vi "clearpath_crio.vi"() -> ()   [LabVIEW 2010]
doc: "Overall demo interface for the cRIO implementation of the Clearpath Control Panel. Allows users to manually issue commands and request subscriptions to a variety of data messages."
uses:
  clearpath_interface.lvlib
panel:
  in  "Int Lim":dbl
  in  "Stic":dbl
  in  "FF":dbl
  in  "D":dbl
  in  "I":dbl
  in  "P":dbl
  in  "Set Controls":bool
  in  "Reset":bool
  in  "Remote E-Stop":bool
  in  "Set Safety":bool
  in  "New Chassis Time (ms)":u32
  in  "Set Time":bool
  in  "New Chassis Name":string
  in  "Set Name":bool
  in  "Max Accel":dbl
  in  "Set Max Accel":bool
  in  "Max Speed":dbl
  in  "Set Max Speed":bool
  in  "Right Accel":dbl
  in  "Left Accel":dbl
  in  "Command Repeat Period (ms)":i32=100
  in  "Continuous Speeds":bool
  in  "Left Speed":dbl
  in  "Right Speed":dbl
  in  "Set Speeds":bool
  in  "Continuous Output":bool
  in  "Left Output":dbl
  in  "Right Output":dbl
  in  "Set Output":bool
  in  "Update Safety Status":bool
  in  "FreqSafetyStatus":u8
  in  "Update Power System":bool
  in  "FreqPowerSystem":u8
  in  "Update Platform Rotation":bool
  in  "FreqPlatformRot":u8
  in  "Update System Status":bool
  in  "FreqSystemStatus":u8
  in  "Update Differential Speed":bool
  in  "FreqDifferentialSpeed":u8
  in  "Update Differential Output":bool
  in  "FreqDifferentialOutput":u8
  in  "Update Differential Control":bool
  in  "FreqDifferentialControl":u8
  in  "Update Platform Name":bool
  in  "FreqPlatformName":u8
  in  "Update Platform Info":bool
  in  "FreqPlatformInfo":u8
  in  "Update Max Accel":bool
  in  "FreqMaxAccel":u8
  in  "Update Max Speed":bool
  in  "FreqMaxSpeed":u8
  in  "Update Firmware Info":bool
  in  "FreqFirmwareInfo":u8
  in  "Update Raw Encoders":bool
  in  "FreqRawEncoder":u8
  in  "Set Brake":bool
  in  "Continuous Vel":bool
  in  "Translational Speed":dbl
  in  "Rotational Speed":dbl
  in  "Set Velocity":bool
  in  "Update Encoder":bool
  in  "FreqEncoder":u8
  in  "VISA resource name":refnum<visa-resource-name>="ASRL1::INSTR"
  in  "Baud rate":dbl=115200.0
  in  "stop":bool
  # "Communication Status"
  # "Subscriptions"
  # "Platform Info (0x8001)"
  # "Differential Control (0x8201)"
  # "Platform Name (0x8002)"
  # "Differential Output (0x8202)"
  # "Firmware Info (0x8003)"
  # "Max Speed (0x8210)"
  # "System Status (0x8004)"
  # "Max Accel (0x8211)"
  # "Power System (0x8005)"
  # "Platform Rotation (0x8601)"
  # "Safety System Status (0x8010)"
  # "Encoders (0x8800)"
  # "Differential Speed (0x8200)"
  # "Raw Encoders (0x8801)"
  # "Set Velocity"
  # "Set Differential Speeds"
  # "Set Chassis Name/Time"
  # "Set Differential Controls"
  # "Set Safety System"
  # "Set Differential Output"
  # "Set Max Speed/Accel"
  # "Reset Processor"
  # "Control Test Panel\nClearpath Control Protocol cRIO Test Interface v1.0\nClearpath Robotics Inc., (c) 2010"
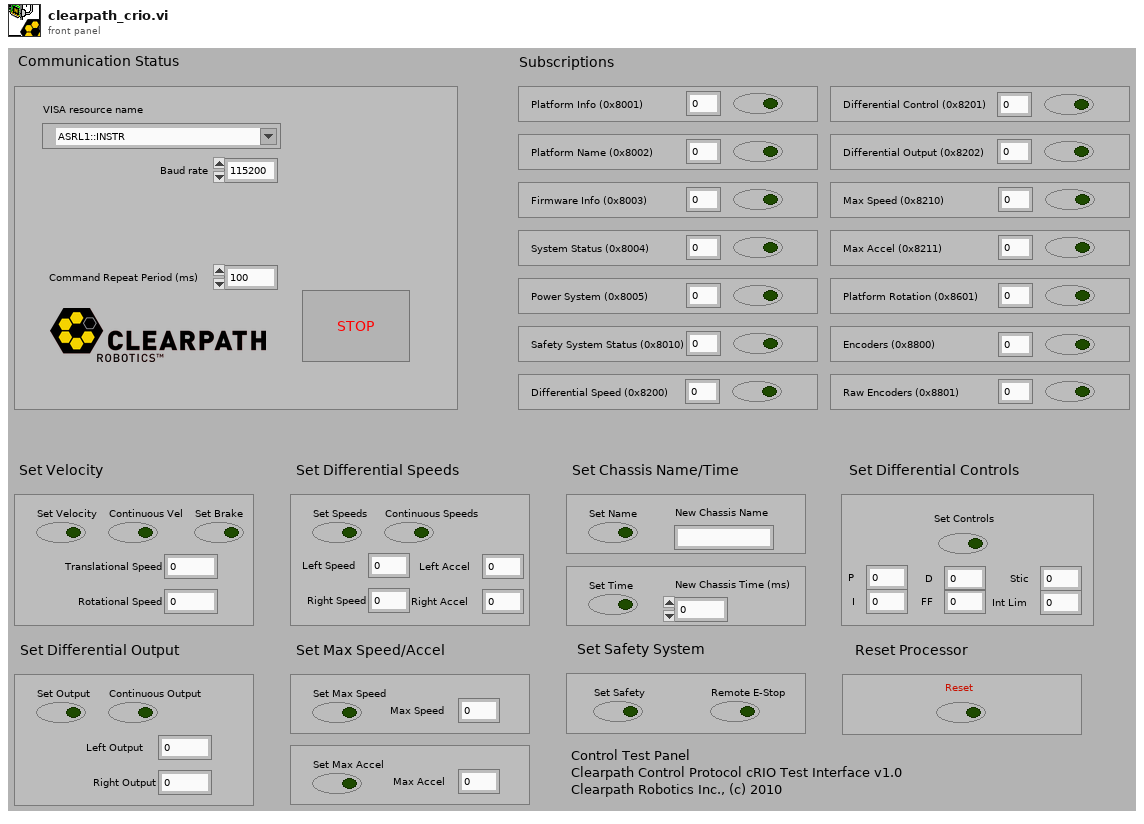
[diagram p1: front panel]
types:
  T1 = cluster{"Xmit Queue":refnum<queue>, "Data Queue":refnum<queue>, "VISA resource name out":refnum<visa-resource-name>, "error out":errorcluster, "Message Data Cluster":cluster{"\nChar Idx":u8, "Num. Char Rem":u8, "Write Index":u8, "Read Index":u8, "Message Data Buffer":u8[][]}}
  T2 = cluster{"P":dbl, "I":dbl, "D":dbl, "FF":dbl, "Stic":dbl, "Int Lim":dbl}
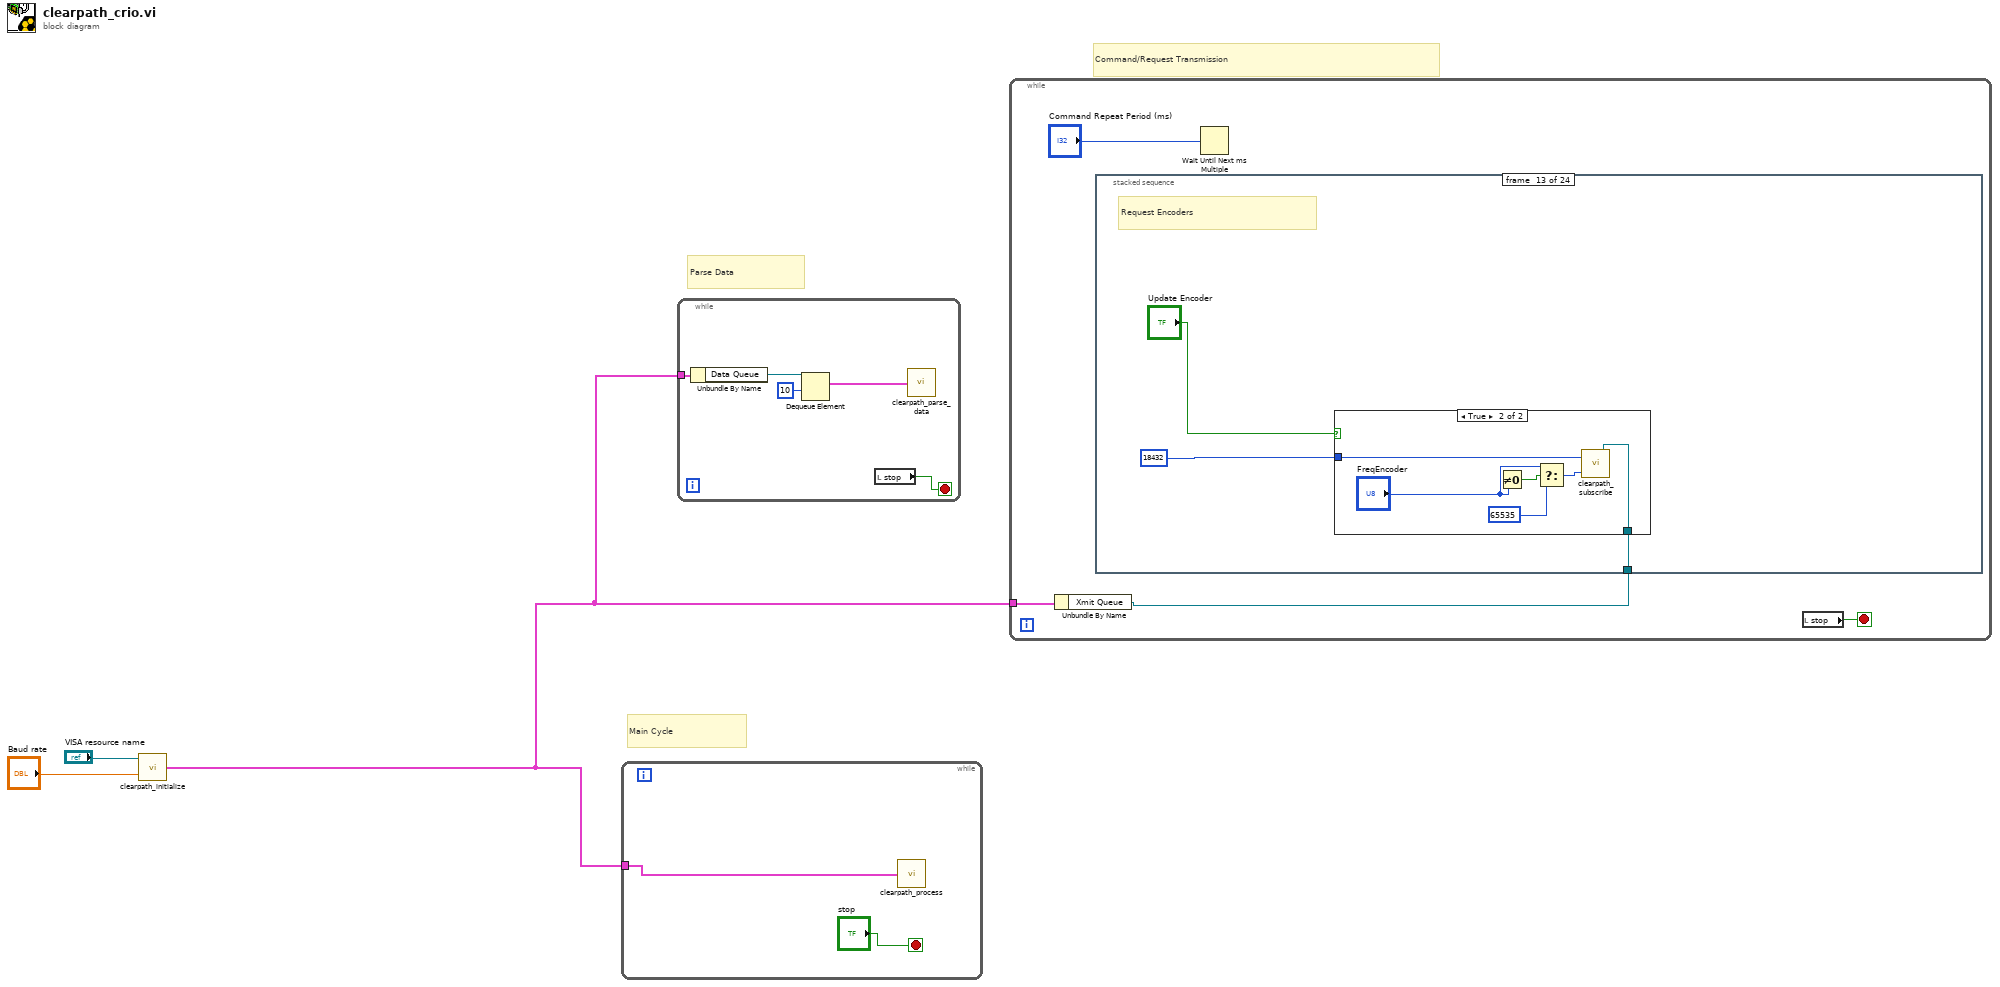
[diagram p0: block diagram]
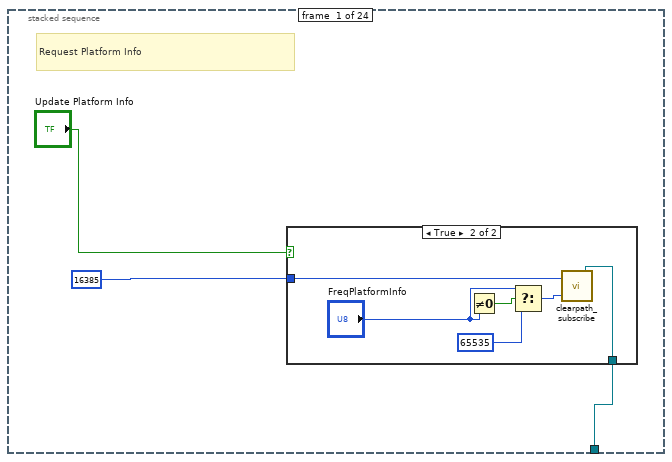
[diagram p2: hidden frame]
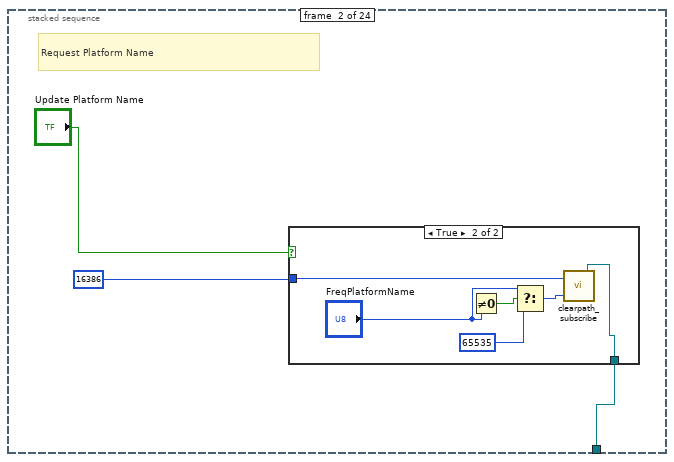
[diagram p4: hidden frame]
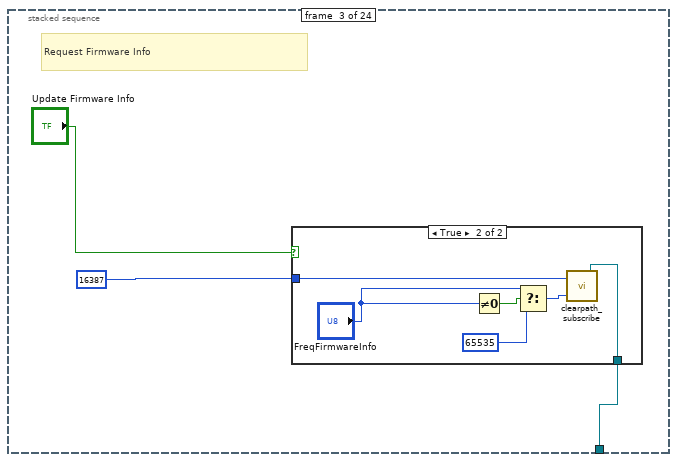
[diagram p6: hidden frame]
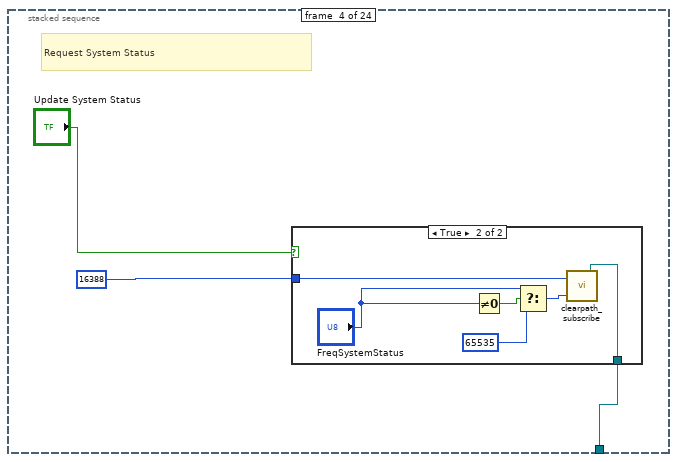
[diagram p8: hidden frame]
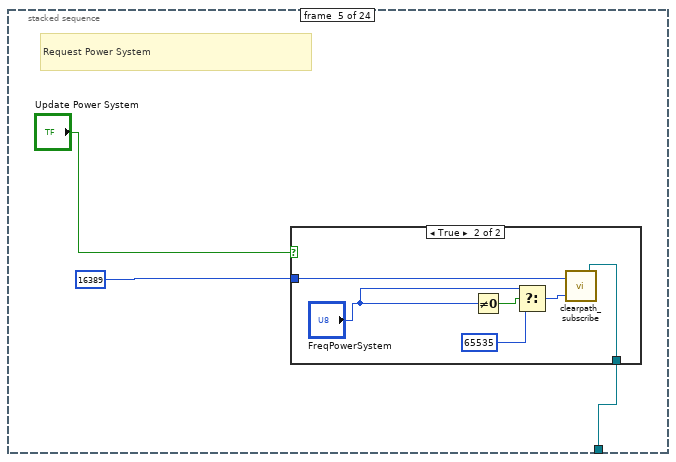
[diagram p10: hidden frame]
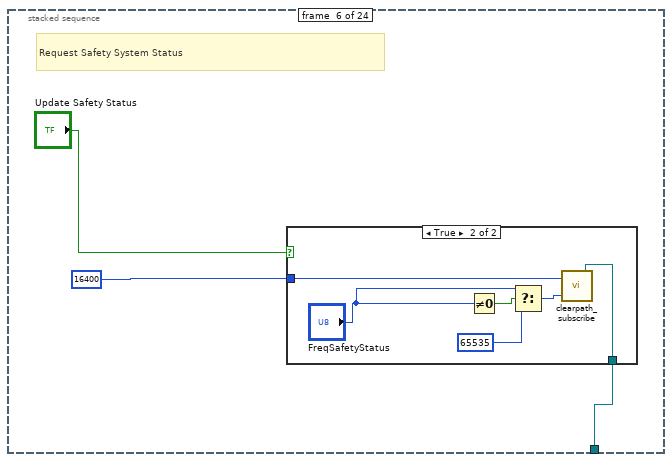
[diagram p12: hidden frame]
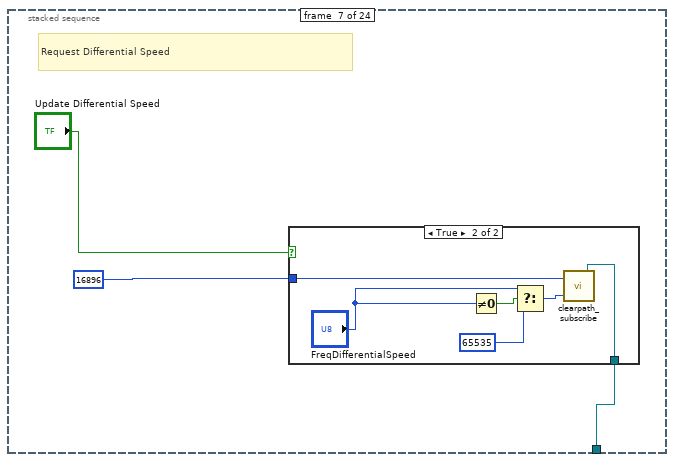
[diagram p14: hidden frame]
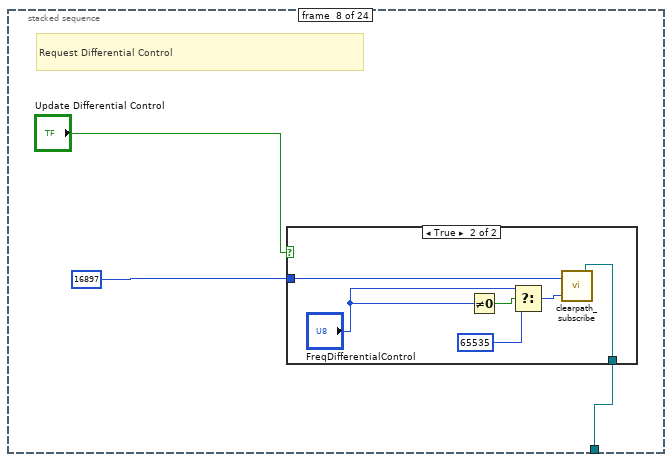
[diagram p16: hidden frame]
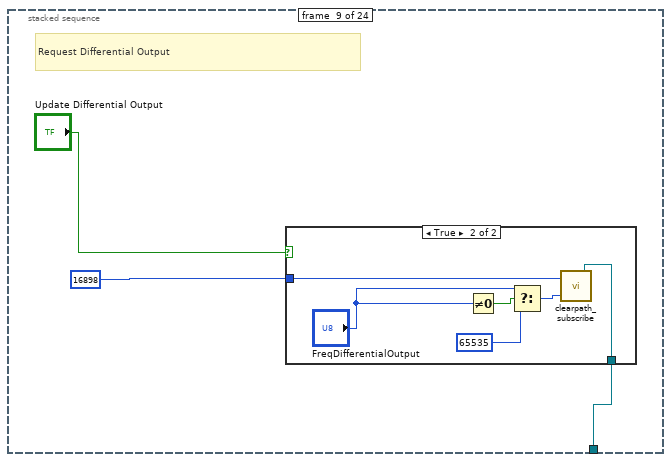
[diagram p18: hidden frame]
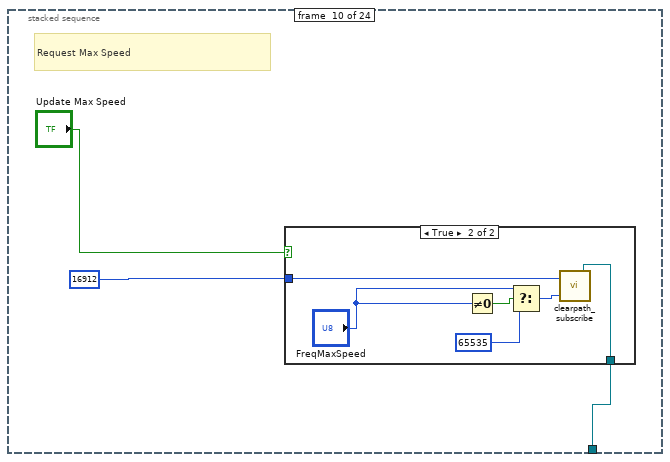
[diagram p20: hidden frame]
diagram:
  # "Main Cycle"
  # "Parse Data"
  # "Command/Request Transmission"
  n1 = call "clearpath_initialize.vi"("Baud rate"="Baud rate", "VISA resource name"="VISA resource name") -> ("Cluster"=w1:T1)
  n2 = while {
    tunnel: w1 -> [w4]
    stop <- "stop" stop-if-true
    n3 = call "clearpath_process.vi"("Clearpath Input"=w4) -> ()
  }
  n4 = while {
    tunnel: w1 -> [w6]
    stop <- w10 stop-if-true
    n5 = Unbundle By Name(w6) -> ("Data Queue"=w7:refnum<queue>)
    n6 = Dequeue Element(queue=w7, timeout in ms (-1)=10) -> (element=w9:cluster{u8[], "Length":i32, "Type":i32})  [unwired: 1 in, 3 out]
    n7 = local read "stop"() -> (w10:bool)
    n8 = call "clearpath_parse_data.vi"("Input Data"=w9) -> ()
  }
  n9 = while {
    tunnel: w1 -> [w11]
    stop <- w14 stop-if-true
    n10 = Unbundle By Name(w11) -> ("Xmit Queue"=w12:refnum<queue>)
    n11 = stacked-sequence {
      tunnel: w12 -> [w16 w26 w34 w43 w52 w61 w70 w79 w88 w97 w106 w116 w125 w134 w142 w146 w150 w155 w162 w173 w179 w186 w190 w194]
      frame #0 {
        # "Request Platform Info"
        n12 = case shown="True" "Update Platform Info" {
          tunnel: w16 -> [_ w18]
          tunnel: 16385 -> [_ w23]
          frame False {
          }
          frame True {
            n13 = Not Equal To 0?(x="FreqPlatformInfo") -> (x != 0?=w21:bool)
            n14 = Select(t="FreqPlatformInfo", s=w21, f=u16 65535) -> (s? t:f=w20:u16)
            n15 = call "clearpath_subscribe.vi"("queue out"=w18, "Frequency"=w20, "Message Type"=w23) -> ()
          }
        }
      }
      frame #1 {
        # "Request Platform Name"
        n16 = case shown="True" "Update Platform Name" {
          tunnel: w26 -> [_ w27]
          tunnel: 16386 -> [_ w32]
          frame False {
          }
          frame True {
            n17 = Not Equal To 0?(x="FreqPlatformName") -> (x != 0?=w30:bool)
            n18 = Select(t="FreqPlatformName", s=w30, f=u16 65535) -> (s? t:f=w29:u16)
            n19 = call "clearpath_subscribe.vi"("queue out"=w27, "Frequency"=w29, "Message Type"=w32) -> ()
          }
        }
      }
      frame #2 {
        # "Request Firmware Info"
        n20 = case shown="True" "Update Firmware Info" {
          tunnel: w34 -> [_ w36]
          tunnel: 16387 -> [_ w41]
          frame False {
          }
          frame True {
            n21 = Not Equal To 0?(x="FreqFirmwareInfo") -> (x != 0?=w39:bool)
            n22 = Select(t="FreqFirmwareInfo", s=w39, f=u16 65535) -> (s? t:f=w38:u16)
            n23 = call "clearpath_subscribe.vi"("queue out"=w36, "Frequency"=w38, "Message Type"=w41) -> ()
          }
        }
      }
      frame #3 {
        # "Request System Status"
        n24 = case shown="True" "Update System Status" {
          tunnel: w43 -> [_ w45]
          tunnel: 16388 -> [_ w50]
          frame False {
          }
          frame True {
            n25 = Not Equal To 0?(x="FreqSystemStatus") -> (x != 0?=w48:bool)
            n26 = Select(t="FreqSystemStatus", s=w48, f=u16 65535) -> (s? t:f=w47:u16)
            n27 = call "clearpath_subscribe.vi"("queue out"=w45, "Frequency"=w47, "Message Type"=w50) -> ()
          }
        }
      }
      frame #4 {
        # "Request Power System"
        n28 = case shown="True" "Update Power System" {
          tunnel: w52 -> [_ w54]
          tunnel: 16389 -> [_ w59]
          frame False {
          }
          frame True {
            n29 = Not Equal To 0?(x="FreqPowerSystem") -> (x != 0?=w57:bool)
            n30 = Select(t="FreqPowerSystem", s=w57, f=u16 65535) -> (s? t:f=w56:u16)
            n31 = call "clearpath_subscribe.vi"("queue out"=w54, "Frequency"=w56, "Message Type"=w59) -> ()
          }
        }
      }
      frame #5 {
        # "Request Safety System Status"
        n32 = case shown="True" "Update Safety Status" {
          tunnel: w61 -> [_ w63]
          tunnel: 16400 -> [_ w68]
          frame False {
          }
          frame True {
            n33 = Not Equal To 0?(x="FreqSafetyStatus") -> (x != 0?=w66:bool)
            n34 = Select(t="FreqSafetyStatus", s=w66, f=u16 65535) -> (s? t:f=w65:u16)
            n35 = call "clearpath_subscribe.vi"("queue out"=w63, "Frequency"=w65, "Message Type"=w68) -> ()
          }
        }
      }
      frame #6 {
        # "Request Differential Speed"
        n36 = case shown="True" "Update Differential Speed" {
          tunnel: w70 -> [_ w72]
          tunnel: 16896 -> [_ w77]
          frame False {
          }
          frame True {
            n37 = Not Equal To 0?(x="FreqDifferentialSpeed") -> (x != 0?=w75:bool)
            n38 = Select(t="FreqDifferentialSpeed", s=w75, f=u16 65535) -> (s? t:f=w74:u16)
            n39 = call "clearpath_subscribe.vi"("queue out"=w72, "Frequency"=w74, "Message Type"=w77) -> ()
          }
        }
      }
      frame #7 {
        # "Request Differential Control"
        n40 = case shown="True" "Update Differential Control" {
          tunnel: w79 -> [_ w81]
          tunnel: 16897 -> [_ w86]
          frame False {
          }
          frame True {
            n41 = Not Equal To 0?(x="FreqDifferentialControl") -> (x != 0?=w84:bool)
            n42 = Select(t="FreqDifferentialControl", s=w84, f=u16 65535) -> (s? t:f=w83:u16)
            n43 = call "clearpath_subscribe.vi"("queue out"=w81, "Frequency"=w83, "Message Type"=w86) -> ()
          }
        }
      }
      frame #8 {
        # "Request Differential Output"
        n44 = case shown="True" "Update Differential Output" {
          tunnel: w88 -> [_ w90]
          tunnel: 16898 -> [_ w95]
          frame False {
          }
          frame True {
            n45 = Not Equal To 0?(x="FreqDifferentialOutput") -> (x != 0?=w93:bool)
            n46 = Select(t="FreqDifferentialOutput", s=w93, f=u16 65535) -> (s? t:f=w92:u16)
            n47 = call "clearpath_subscribe.vi"("queue out"=w90, "Frequency"=w92, "Message Type"=w95) -> ()
          }
        }
      }
      frame #9 {
        # "Request Max Speed"
        n48 = case shown="True" "Update Max Speed" {
          tunnel: w97 -> [_ w99]
          tunnel: 16912 -> [_ w104]
          frame False {
          }
          frame True {
            n49 = Not Equal To 0?(x="FreqMaxSpeed") -> (x != 0?=w102:bool)
            n50 = Select(t="FreqMaxSpeed", s=w102, f=u16 65535) -> (s? t:f=w101:u16)
            n51 = call "clearpath_subscribe.vi"("queue out"=w99, "Frequency"=w101, "Message Type"=w104) -> ()
          }
        }
      }
      frame #10 {
        # "Request Max Accel"
        n52 = case shown="True" "Update Max Accel" {
          tunnel: w106 -> [_ w108]
          tunnel: 16913 -> [_ w113]
          frame False {
          }
          frame True {
            n53 = Not Equal To 0?(x="FreqMaxAccel") -> (x != 0?=w111:bool)
            n54 = Select(t="FreqMaxAccel", s=w111, f=u16 65535) -> (s? t:f=w110:u16)
            n55 = call "clearpath_subscribe.vi"("queue out"=w108, "Frequency"=w110, "Message Type"=w113) -> ()
          }
        }
      }
      frame #11 {
        # "Request Platform Rotation"
        n56 = case shown="True" "Update Platform Rotation" {
          tunnel: w116 -> [_ w117]
          tunnel: 17921 -> [_ w122]
          frame False {
          }
          frame True {
            n57 = Not Equal To 0?(x="FreqPlatformRot") -> (x != 0?=w120:bool)
            n58 = Select(t="FreqPlatformRot", s=w120, f=u16 65535) -> (s? t:f=w119:u16)
            n59 = call "clearpath_subscribe.vi"("queue out"=w117, "Frequency"=w119, "Message Type"=w122) -> ()
          }
        }
      }
      frame #12 {
        # "Request Encoders"
        n60 = case shown="True" "Update Encoder" {
          tunnel: w125 -> [_ w126]
          tunnel: 18432 -> [_ w131]
          frame False {
          }
          frame True {
            n61 = Not Equal To 0?(x="FreqEncoder") -> (x != 0?=w128:bool)
            n62 = Select(t="FreqEncoder", s=w128, f=u16 65535) -> (s? t:f=w127:u16)
            n63 = call "clearpath_subscribe.vi"("queue out"=w126, "Frequency"=w127, "Message Type"=w131) -> ()
          }
        }
      }
      frame #13 {
        # "Request Raw Encoders"
        n64 = case shown="True" "Update Raw Encoders" {
          tunnel: w134 -> [_ w135]
          tunnel: 18433 -> [_ w140]
          frame False {
          }
          frame True {
            n65 = Not Equal To 0?(x="FreqRawEncoder") -> (x != 0?=w138:bool)
            n66 = Select(t="FreqRawEncoder", s=w138, f=u16 65535) -> (s? t:f=w137:u16)
            n67 = call "clearpath_subscribe.vi"("queue out"=w135, "Frequency"=w137, "Message Type"=w140) -> ()
          }
        }
      }
      frame #14 {
        # "Set Platform Name"
        n68 = case shown="True" "Set Name" {
          tunnel: w142 -> [_ w143]
          frame False {
          }
          frame True {
            n69 = call "clearpath_set_platform_name.vi"("queue out"=w143, "New Name"="New Chassis Name") -> ()
          }
        }
      }
      frame #15 {
        # "Set Platform Time"
        n70 = case shown="True" "Set Time" {
          tunnel: w146 -> [_ w147]
          frame False {
          }
          frame True {
            n71 = call "clearpath_set_platform_time.vi"("queue out"=w147, "New Time"="New Chassis Time (ms)") -> ()
          }
        }
      }
      frame #16 {
        # "Set Safety System"
        n72 = case shown="True" "Set Safety" {
          tunnel: w150 -> [_ _]
          frame False {
          }
          frame True {
            n73 = call "clearpath_set_safety_system.vi"("Set Stop Flag"="Remote E-Stop") -> ()  [unwired: 1 in]
          }
        }
      }
      frame #17 {
        # "Set Differential Speeds"
        n74 = Or(x="Continuous Speeds", y="Set Speeds") -> (x .or. y?=w153:bool)
        n75 = case shown="True" w153 {
          tunnel: w155 -> [_ w156]
          frame False {
          }
          frame True {
            n76 = call "clearpath_set_differential_speeds.vi"("queue out"=w156, "Right Accel"="Right Accel", "Left Accel"="Left Accel", "Right Speed"="Right Speed", "Left Speed"="Left Speed") -> ()
          }
        }
      }
      frame #18 {
        # "Set Differential Controls"
        n77 = case shown="True" "Set Controls" {
          tunnel: w162 -> [_ _]
          frame False {
          }
          frame True {
            n78 = Bundle("P"="P", "I"="I", "D"="D", "FF"="FF", "Stic"="Stic", "Int Lim"="Int Lim") -> (w163:T2)  [unwired: 1 in]
            n79 = call "clearpath_set_differential_controls.vi"("Controls Cluster"=w163) -> ()  [unwired: 1 in]
          }
        }
      }
      frame #19 {
        # "Set Differential Output"
        n80 = Or(x="Continuous Output", y="Set Output") -> (x .or. y?=w171:bool)
        n81 = case shown="True" w171 {
          tunnel: w173 -> [_ w174]
          frame False {
          }
          frame True {
            n82 = call "clearpath_set_differential_output.vi"("queue out"=w174, "Right Output"="Right Output", "Left Output"="Left Output") -> ()
          }
        }
      }
      frame #20 {
        # "Set Velocity"
        n83 = Or(x="Continuous Vel", y="Set Velocity") -> (x .or. y?=w178:bool)
        n84 = case shown="True" w178 {
          tunnel: w179 -> [_ w181]
          frame False {
          }
          frame True {
            n85 = call "clearpath_set_velocity.vi"("queue out"=w181, "Zero Speeds"="Set Brake", "Rotational Speed"="Rotational Speed", "Translational Speed"="Translational Speed") -> ()
          }
        }
      }
      frame #21 {
        # "Set Max Speed"
        n86 = case shown="True" "Set Max Speed" {
          tunnel: w186 -> [_ w187]
          frame False {
          }
          frame True {
            n87 = call "clearpath_set_max_speed.vi"("queue out"=w187, "Max Speed"="Max Speed") -> ()
          }
        }
      }
      frame #22 {
        # "Set Max Accel"
        n88 = case shown="True" "Set Max Accel" {
          tunnel: w190 -> [_ w191]
          frame False {
          }
          frame True {
            n89 = call "clearpath_set_max_accel.vi"("queue out"=w191, "Max Accel"="Max Accel") -> ()
          }
        }
      }
      frame #23 {
        # "Reset Processor"
        n90 = case shown="True" "Reset" {
          tunnel: w194 -> [_ w195]
          frame False {
          }
          frame True {
            n91 = call "clearpath_set_reset.vi"("queue out"=w195) -> ()
          }
        }
      }
    }
    n92 = Wait Until Next ms Multiple(millisecond multiple="Command Repeat Period (ms)") -> ()  [unwired: 1 out]
    n93 = local read "stop"() -> (w14:bool)
  }
